vi "X_IMAQ Convert Point to ROI.vi"(7 "error in (no error)":errorcluster, 10 "Point":T2 {"Y" format="%.2f"; "X" format="%.2f"}) -> (0 "error out":errorcluster, 3 "ROI Descriptor":T1 {"Contours"."Type" items=["No Selection", "Point", "Line", "Rectangle", "Oval", "Polygon", "Freehand Region", "Annulus", "Unused2", "Unused3", "Broken Line", "Freehand Line", "Rotated Rectangle"]})   [LabVIEW 2021, in "Image.lvlib"]
doc: "Converts a point element to an ROI Descriptor."
uses:
  Image.lvlib
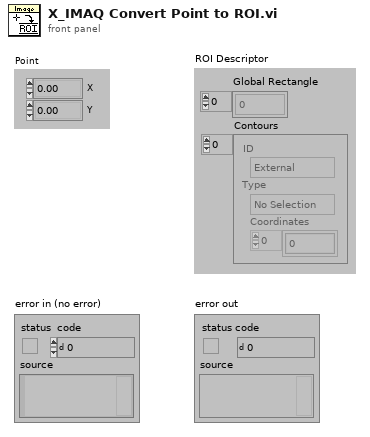
[diagram p1: front panel]
types:
  T1 = typedef "ROI Descriptor" = cluster{"Global Rectangle":i32[], "Contours":cluster{"ID":enum32{"External", "Internal"}, "Type":u32, "Coordinates":i32[]}[]}
  T2 = typedef "IMAQ Point" = cluster{"X":sgl, "Y":sgl}
  T3 = cluster{"ID":enum32{"External", "Internal"}, "Type":u32, i32[]}
  T4 = cluster{"ID":enum32{"External", "Internal"}, "Type":u32, i32[]}[]
  T5 = cluster{i32[], cluster{"ID":enum32{"External", "Internal"}, "Type":u32, i32[]}[]}
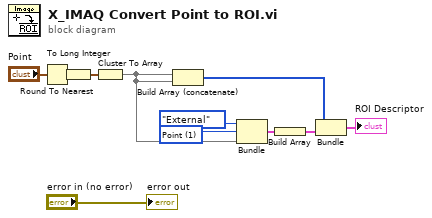
[diagram p0: block diagram]
diagram:
  w8 = u32 1 items=["No Selection", "Point", "Line", "Rectangle", "Oval", "Polygon", "Free", "Annulus", "Unused2", "Unused3", "Broken Line", "Free Hand Line", "Rotated Rectangle"] ("Type")
  n1 = Round To Nearest(number="Point") -> (nearest integer value=w6:T2)
  n2 = To Long Integer(number=w6) -> (32bit integer=w5:cluster{"X":i32, "Y":i32})
  n3 = Cluster To Array(cluster=w5) -> (array=w1:i32[])
  n4 = Build Array (concatenate)(w1, w1) -> (w4:i32[])
  n5 = Bundle("ID"=enum32{"External", "Internal"}."External", "Type"=w8, w1) -> (w10:T3)  [unwired: 1 in]
  n6 = Build Array(w10) -> (w11:T4)
  n7 = Bundle(w4, w11) -> (→"ROI Descriptor":T5)  [unwired: 1 in]
  "error out" <- "error in (no error)"
